vi "Flyout.vi"(8 "error in (no error)":errorcluster, 9 "Message Queue":refnum<queue>, 10 "Timeout":dbl, 11 "Message":string) -> (0 "error out":errorcluster)   [LabVIEW 2019, in "Flyout.lvlib"]
uses:
  Flyout.lvlib
  MainController/Cluster - MainControllerMessage.ctl
  MainController/Enum - MainState.ctl
  MainController/MainController.lvlib
panel:
  out "MessageDisplay":string
  in  "Close":bool
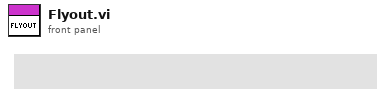
[diagram p1: front panel]
types:
  T1 = typedef "MainController.lvlib/Enum - MainState.ctl" = enum16{"Initialize", "InitUIRefs", "LaunchSettings", "LaunchAutoMode", "LaunchManualMode", "LaunchTestReport", "ConnectHardware", "DisconnectHardware", "HiliteNavItems", "StartAutoMode", "PauseAutoMode", "StopAutoMode", "ShowFlyout", "HideFlyout", "BroadcastSettings", "PickupTestSettings", "BroadcastHW", "AutoTestDone", "DAQStatus", "UpdateCommandBar", "Error", "RecieveError", "Exit"}
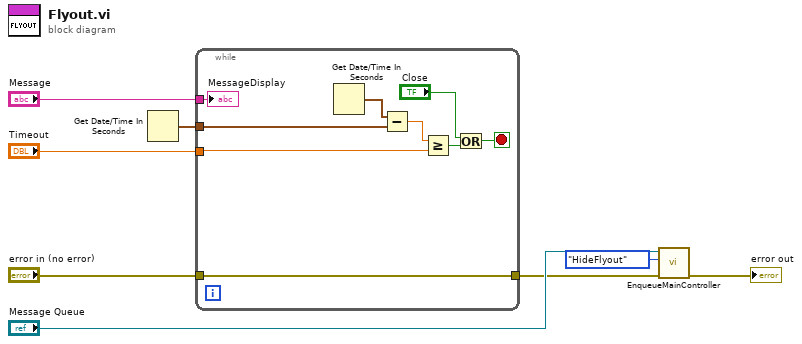
[diagram p0: block diagram]
diagram:
  n1 = Get Date/Time In Seconds() -> (seconds since 1Jan1904=w7:timestamp)
  n2 = while {
    tunnel: "Timeout" -> [w14]
    tunnel: w7 -> [w16]
    tunnel: [w10] -> w4
    tunnel: "error in (no error)" -> [w10]
    tunnel: "Message" -> [w9]
    stop <- w12 stop-if-true
    n3 = Get Date/Time In Seconds() -> (seconds since 1Jan1904=w17:timestamp)
    n4 = Subtract(x=w17, y=w16) -> (x-y=w15:dbl)
    n5 = Greater Or Equal?(x=w15, y=w14) -> (x >= y?=w13:bool)
    n6 = Or(x="Close", y=w13) -> (x .or. y?=w12:bool)
    "MessageDisplay" <- w9
  }
  n7 = call "EnqueueMainController.vi"("error in (no error)"=w4, "Message"=Enum_-_MainState."HideFlyout", "MainQueue"="Message Queue") -> ("error out"=→"error out":errorcluster)  [unwired: 6 in, 2 out]
